vi "Valid.vi"(11 "Parallel Process in":refnum<class "Parallel Process.lvclass">) -> (2 "Valid?":bool, 3 "Parallel Process out":refnum<class "Parallel Process.lvclass">)   [LabVIEW 2011, in "Messenging.lvlib" / "Parallel Process.lvclass"]
uses:
  Parallel Process.lvclass
  Parallel Process.lvclass/Parallel Process.ctl
  Interprocess Messenger/Messenger (Parent)/MGR.lvclass
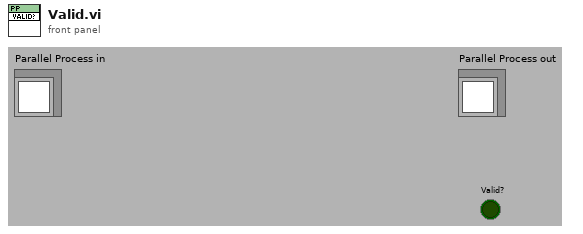
[diagram p1: front panel]
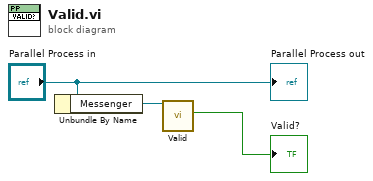
[diagram p0: block diagram]
diagram:
  n1 = Unbundle By Name("Parallel Process in") -> ("Messenger"=w2:refnum<class "MGR.lvclass">)
  n2 = call-dynamic "Valid.vi"("Send in"=w2) -> ("Valid?"=→"Valid?":bool)  [unwired: 10 out]
  "Parallel Process out" <- "Parallel Process in"
